vi "Race Random Numbers.vi"() -> ()   [LabVIEW 2014]
doc: "This VI uses 2 random number generators and sums their results. The user tells the VI how many bits the numbers that are generated should be, and specifies a total for the sum."
uses:
  <vilib>/imath/engines/lvmath2/RunTimeEngine/Managers/WorkSpace/UID Generator.vi
  <vilib>/imath/engines/lvmath2/RunTimeEngine/RunTimeType/NIMS_RunTimeType_From StrictType (excl LVString).vi
  <instcachedir>/0/NIMS_RunTimeType_From StrictType (excl LVString)_15A5391EEA9C4AACB9955AC755B83D29.lvgen/NIMS_RunTimeType_From StrictType (excl LVString)_15A5391EEA9C4AACB9955AC755B83D29_000.vi
  <vilib>/imath/engines/lvmath2/RunTimeEngine/LocalVariableDefStatement/MC_LocalVariableDefStatement_Display.vi
  <vilib>/imath/engines/lvmath2/RunTimeEngine/Managers/SymbolTable/Clear UID.vi
  <vilib>/imath/engines/lvmath2/RunTimeEngine/NodeEndStatement/NIMS_NodeEndStatement_Output.vi
  <instcachedir>/0/NIMS_NodeEndStatement_Output_53EC0D466D134D7ABD903AC30B43404B.lvgen/NIMS_NodeEndStatement_Output_53EC0D466D134D7ABD903AC30B43404B_012.vi
  <vilib>/imath/engines/lvmath2/RunTimeEngine/ErrorHandling/NIMS_Finalize Error.vi
  <vilib>/imath/engines/lvmath2/RunTimeEngine/Managers/SymbolTable/NIMS_WorkSpace.lvlib
panel:
  out "Total Numbers Generated per Generator":i32
  out "?":bool
  out "?":bool
  out "Generator 2":i32
  out "Generator 1":i32
  out "Sum":i32[][](graph)=[[0], [1]]
  in  "Final Number":i32=10
  in  "Number of Bits":i32=2
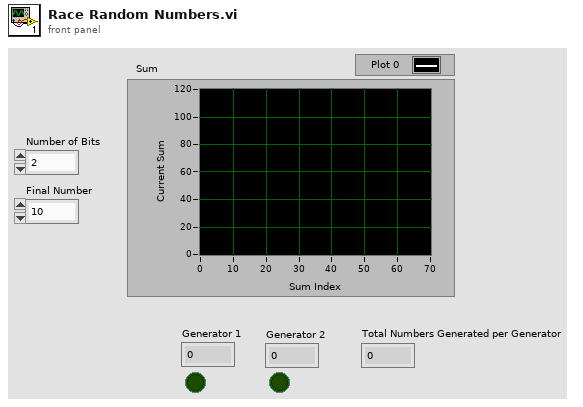
[diagram p1: front panel]
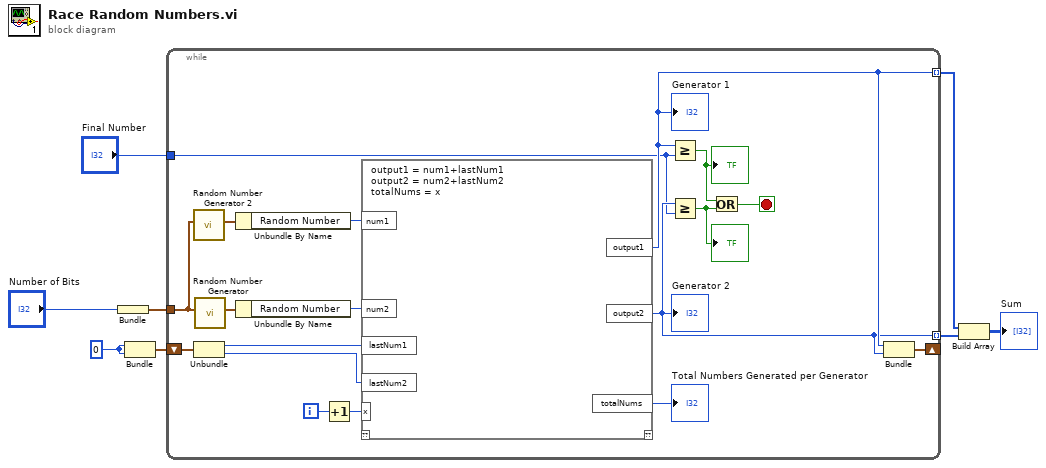
[diagram p0: block diagram]
diagram:
  w6 = 0
  n1 = Bundle("Number of Bits"="Number of Bits") -> (w7:cluster{"Number of Bits":i32})  [unwired: 1 in]
  n2 = Bundle(w6, w6) -> (w5:cluster{i32, i32})  [unwired: 1 in]
  n3 = while {
    tunnel: w7 -> [w26]
    shift-right: [w18] -> _
    shift-left: w5 -> [w21]
    tunnel: [w17] -> w4 mode=indexing
    tunnel: [w16] -> w3 mode=indexing
    tunnel: "Final Number" -> [w14]
    i -> [w10]
    stop <- w15 stop-if-true
    n4 = call "Random Number Generator 2.vi"("Binary Digits"=w26) -> ("Random Number"=w25:cluster{"Random Number":i32})  [unwired: 10 in]
    n5 = Unbundle(w21) -> (w20:i32, w19:i32)
    n6 = call "Random Number Generator.vi"("Binary Digits"=w26) -> ("Random Number"=w22:cluster{"Random Number":i32})  [unwired: 10 in]
    n7 = Unbundle By Name(w25) -> ("Random Number"=w24:i32)
    n8 = Unbundle By Name(w22) -> ("Random Number"=w23:i32)
    n9 = Increment(x=w10) -> (x+1=w9:i32)
    n10 = mathscript code="output1 = num1+lastNum1\noutput2 = num2+lastNum2\ntotalNums = x"("num1"=w24, "num2"=w23, "lastNum1"=w20, "lastNum2"=w19, "x"=w9) -> ("output1"=w17:i32, "output2"=w16:i32, "totalNums"=→"Total Numbers Generated per Generator":i32)  [unwired: 1 in, 1 out]
    "Generator 1" <- w17
    "Generator 2" <- w16
    n11 = Greater Or Equal?(x=w17, y=w14) -> (x >= y?=w12:bool)
    "?" <- w12
    n12 = Greater Or Equal?(x=w16, y=w14) -> (x >= y?=w13:bool)
    "?" <- w13
    n13 = Or(x=w12, y=w13) -> (x .or. y?=w15:bool)
    n14 = Bundle("output1"=w17, "output2"=w16) -> (w18:cluster{"output1":i32, "output2":i32})  [unwired: 1 in]
  }
  n15 = Build Array(w4, w3) -> (→"Sum":i32[][])
